vi "CoreVideo.vi"(11 "Cluster":T1) -> ()   [LabVIEW 2024]
uses:
  dacAquisition/#AquisitionLoopEnum.ctl
  <vilib>/vision/driver/IMAQdx.llb/IMAQdx Camera Control Mode.ctl
  <vilib>/vision/driver/NI_Vision_Acquisition_Software.lvlib
  <vilib>/vision/Image Controls.llb/IMAQ Image.ctl
  #VideoQueueElement.ctl
  #VisionProcessingEnum.ctl
  GUI/#GuiEnum.ctl
  GUI/#GuiQueueElement.ctl
  #QueueEnum.ctl
  Correlation/#CorrelationQueueElement.ctl
  <vilib>/userDefined/High Color/IMAQdx.ctl
  Core/#CoreQueues.ctl
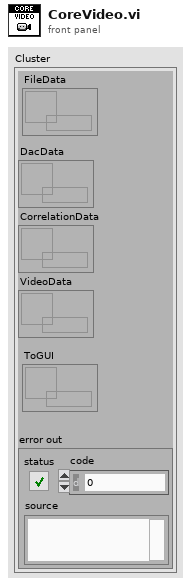
[diagram p1: front panel]
types:
  T1 = typedef "#CoreQueues.ctl" = cluster{"DacData":refnum<queue>, "CorrelationData":refnum<queue>, "VideoData":refnum<queue>, "error out":errorcluster, "ToGUI":refnum<queue>, "FileData":refnum<queue>}
  T2 = typedef "IMAQ Image.ctl" = refnum<image>
  T3 = typedef "IMAQdx.ctl" = refnum<k21>
  T4 = typedef "Image Type" = u32
  T5 = typedef "#VisionProcessingEnum.ctl" = enum16{"Init", "Processing", "ProcessingVision", "Close"}
  T6 = typedef "#AquisitionLoopEnum.ctl" = enum16{"Idle", "Init", "Aquisition", "End"}
  T7 = typedef "NI_Vision_Acquisition_Software.lvlib/IMAQdx Camera Control Mode.ctl" = enum32{"Controller", "Listener"}
  T8 = typedef "#VideoQueueElement.ctl" = cluster{"Image Out":T2, "current time":timestamp}
  T9 = typedef "#AntennaControlNumber.ctl" = enum16{"Ant1", "Ant2", "Ant3", "Ant4"}
  T10 = cluster{"Reverse fingers":bool, "SelectingButton":bool, "Antenna":T9, "TestVsion":bool, "Camera source":T3, "AntDistance [mm]":dbl}
  T11 = typedef "#GuiEnum.ctl" = enum16{"AudioData", "VisionDistances", "DacDistances", "CorrelationDistances", "Video", "FPS"}
  T12 = typedef "#GuiQueueElement.ctl" = cluster{"Enum":T11, "Variant":variant}
  T13 = typedef "#QueueEnum.ctl" = enum16{"Ant", "Video"}
  T14 = typedef "#CorrelationQueueElement.ctl" = cluster{"Enum":T13, "t0":timestamp, dbl[]}
  T15 = cluster{"Image Out":T2, "current time":timestamp}
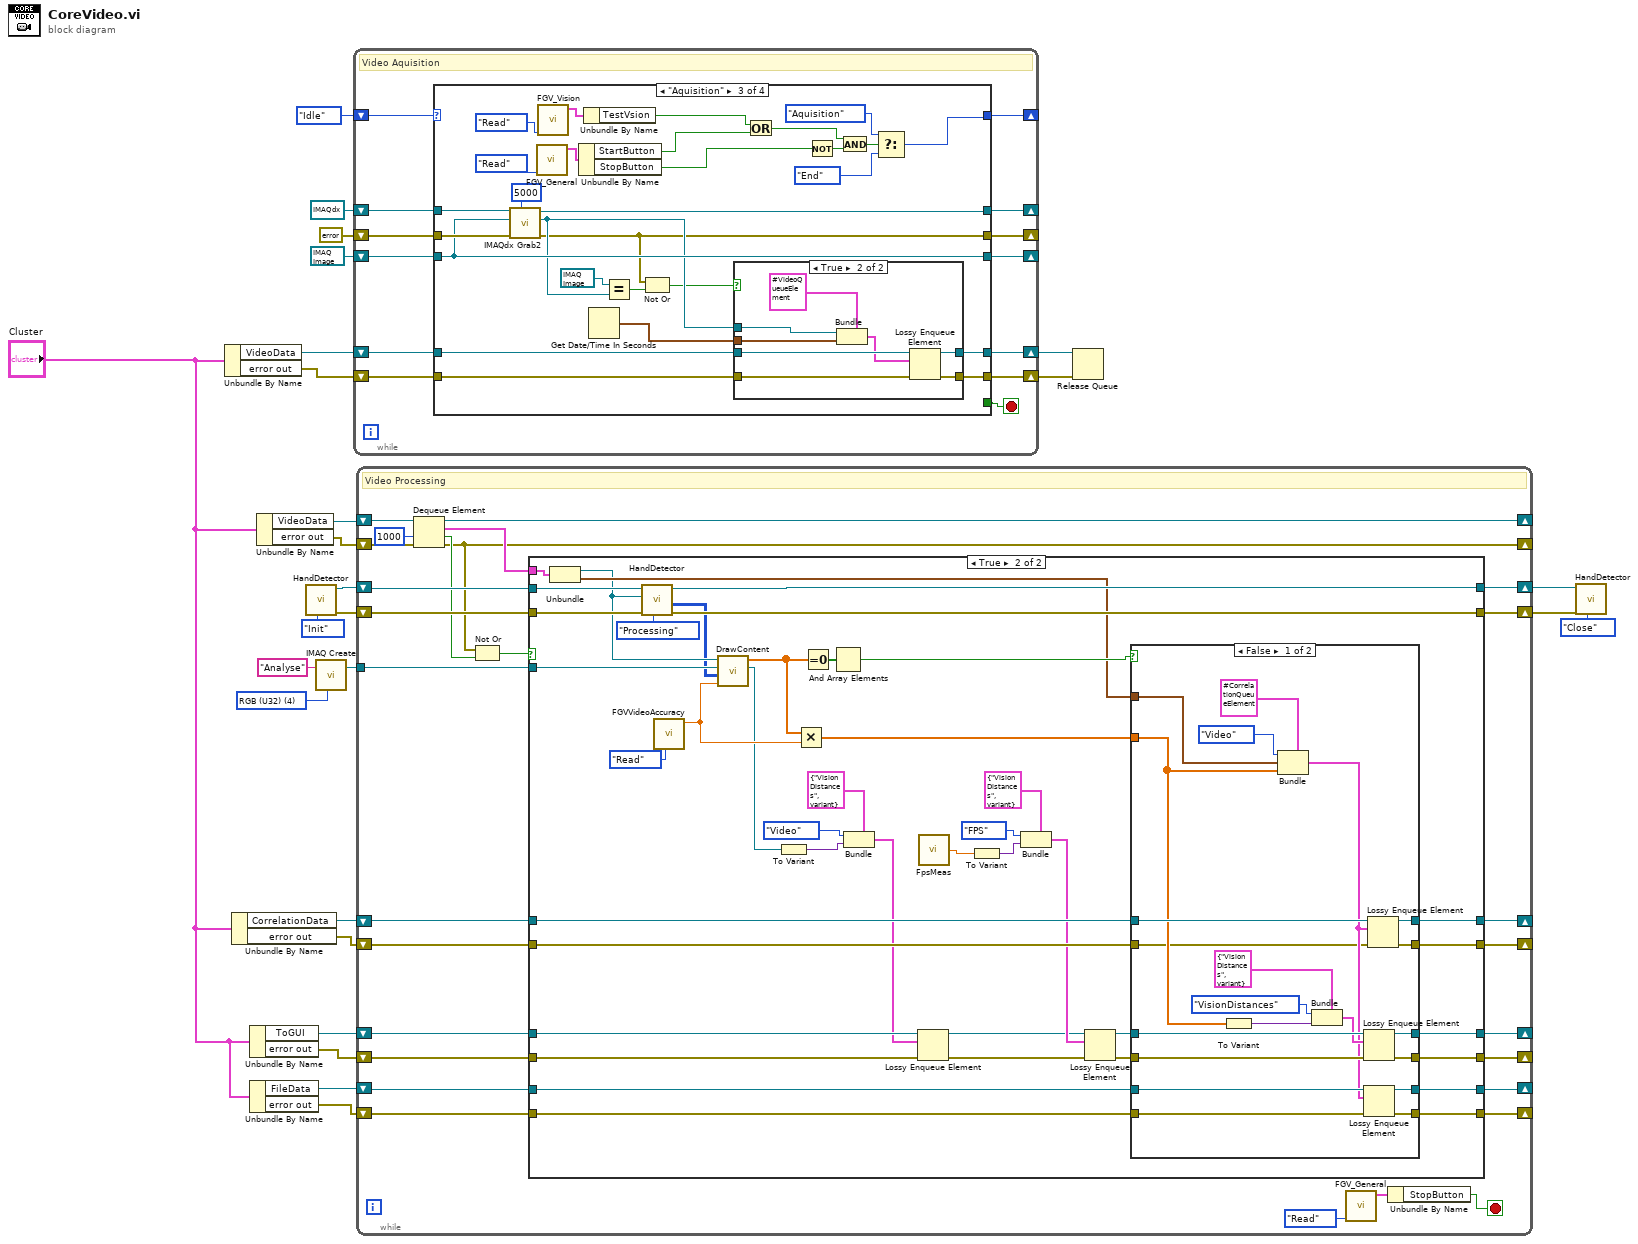
[diagram p0: block diagram]
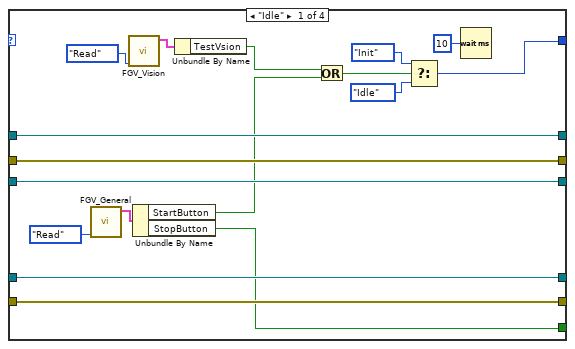
[diagram p4: hidden frame]
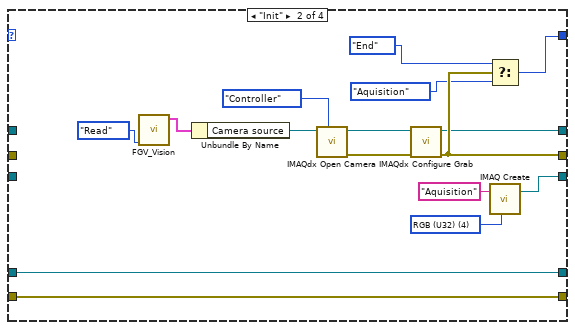
[diagram p5: hidden frame]
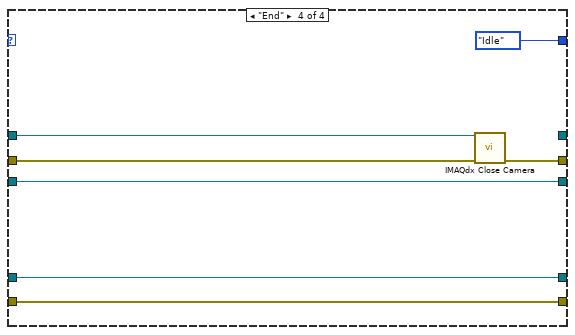
[diagram p7: hidden frame]
diagram:
  w12 = T4 4 items=["Grayscale (U8)", "Grayscale (I16)", "Grayscale (SGL)", "Complex (CSG)", "RGB (U32)", "HSL (U32)", "RGB (U64)", "Grayscale (U16)"] ("Image Type")
  n1 = Unbundle By Name("Cluster") -> ("VideoData"=w16:refnum<queue>, "error out"=w17:errorcluster)
  n2 = Unbundle By Name("Cluster") -> ("CorrelationData"=w23:refnum<queue>, "error out"=w24:errorcluster)
  n3 = Unbundle By Name("Cluster") -> ("ToGUI"=w25:refnum<queue>, "error out"=w26:errorcluster)
  n4 = Unbundle By Name("Cluster") -> ("FileData"=w3:refnum<queue>, "error out"=w2:errorcluster)
  n5 = Unbundle By Name("Cluster") -> ("VideoData"=w21:refnum<queue>, "error out"=w22:errorcluster)
  n6 = call "HandDetector.vi"("Enum"=#VisionProcessingEnum."Init") -> ("error out"=w10:errorcluster, "session out"=w9:refnum<k35>)  [unwired: 6 in, 3 out]
  n7 = call "IMAQ Create"("Image Name"="Analyse", "Image Type"=w12) -> ("New Image"=w13:T2)  [unwired: 3 in, 1 out]
  n8 = while {
    shift-right: [w39] -> _
    shift-left: T3 refnum ("Session Out") -> [w36]
    shift-right: [w38] -> _
    shift-left: errorcluster {"status"=FALSE, "code"=0, "source"=""} ("error out") -> [w37]
    shift-right: [w34] -> _
    shift-left: #AquisitionLoopEnum."Idle" -> [w35]
    shift-right: [w33] -> w14
    shift-left: w16 -> [w30]
    shift-right: [w32] -> w15
    shift-left: w17 -> [w31]
    shift-right: [w29] -> _
    shift-left: T2 refnum ("New Image") -> [w28]
    stop <- w27 stop-if-true
    # "Video Aquisition"
    n9 = case shown="\"Aquisition\"" w35 {
      tunnel: [w56 w57 w73 _] -> w39
      tunnel: [w55 w64 w83 w116] -> w38
      tunnel: w37 -> [w55 _ w100 w117]
      tunnel: w36 -> [w56 _ w74 w111]
      tunnel: [w51 w61 w94 #AquisitionLoopEnum."Idle"] -> w34
      tunnel: [w48 w69 w92 w114] -> w33
      tunnel: [w49 w68 w91 w113] -> w32
      tunnel: w31 -> [w49 w68 w90 w113]
      tunnel: w30 -> [w48 w69 w89 w114]
      tunnel: [w47 w67 w88 w112] -> w29
      tunnel: w28 -> [w47 _ w88 w112]
      tunnel: [w44 _ _ _] -> w27
      frame "Idle" {
        n10 = call "FGV_General.vi"("Type"=enum16{"Read", "Write"}."Read") -> ("GeneralIndicator"=w45:cluster{"StartButton":bool, "StopButton":bool})  [unwired: 10 in]
        n11 = call "FGV_Vision.vi"("Operation"=enum16{"Read", "Write"}."Read") -> ("OutVision"=w41:T10)  [unwired: 8 in]
        n12 = Unbundle By Name(w45) -> ("StartButton"=w43:bool, "StopButton"=w44:bool)
        n13 = Unbundle By Name(w41) -> ("TestVsion"=w40:bool)
        n14 = Or(x=w40, y=w43) -> (x .or. y?=w54:bool)
        n15 = Select(t=#AquisitionLoopEnum."Init", s=w54, f=#AquisitionLoopEnum."Idle") -> (s? t:f=w51:T6)
        n16 = Wait (ms)(milliseconds to wait=u32 10) -> ()  [unwired: 1 out]
      }
      frame "Init" {
        w65 = T4 4 items=["Grayscale (U8)", "Grayscale (I16)", "Grayscale (SGL)", "Complex (CSG)", "RGB (U32)", "HSL (U32)", "RGB (U64)", "Grayscale (U16)"] ("Image Type")
        n17 = call "FGV_Vision.vi"("Operation"=enum16{"Read", "Write"}."Read") -> ("OutVision"=w59:T10)  [unwired: 8 in]
        n18 = Unbundle By Name(w59) -> ("Camera source"=w58:T3)
        n19 = call <vilib>:"IMAQdx Open Camera.vi"("Camera Control Mode"=IMAQdx_Camera_Control_Mode."Controller", "Session In"=w58) -> ("error out"=w70:errorcluster, "Session Out"=w72:T3)  [unwired: 8 in]
        n20 = call <vilib>:"IMAQdx Configure Grab.vi"("error in"=w70, "Session In"=w72) -> ("error out"=w64:errorcluster, "Session Out"=w57:T3)  [unwired: 8 in]
        n21 = Select(t=#AquisitionLoopEnum."End", s=w64, f=#AquisitionLoopEnum."Aquisition") -> (s? t:f=w61:T6)
        n22 = call "IMAQ Create"("Image Name"="Aquisition", "Image Type"=w65) -> ("New Image"=w67:T2)  [unwired: 3 in, 1 out]
      }
      frame "Aquisition" {
        n23 = call <vilib>:"IMAQdx Grab2.vi"("Timeout (ms)"=5000, "error in"=w100, "Image In"=w88, "Session In"=w74) -> ("error out"=w83:errorcluster, "Image Out"=w86:T2, "Session Out"=w73:T3)  [unwired: 4 in, 1 out]
        n24 = call "FGV_General.vi"("Type"=enum16{"Read", "Write"}."Read") -> ("GeneralIndicator"=w80:cluster{"StartButton":bool, "StopButton":bool})  [unwired: 10 in]
        n25 = call "FGV_Vision.vi"("Operation"=enum16{"Read", "Write"}."Read") -> ("OutVision"=w76:T10)  [unwired: 8 in]
        n26 = Unbundle By Name(w80) -> ("StartButton"=w78:bool, "StopButton"=w79:bool)
        n27 = Unbundle By Name(w76) -> ("TestVsion"=w75:bool)
        n28 = Get Date/Time In Seconds() -> (seconds since 1Jan1904=w82:timestamp)
        n29 = Equal?(x=T2 refnum ("Image Out"), y=w86) -> (x = y?=w84:bool)
        n30 = Not Or(1:w84, 2:w83) -> (0:w85:bool)
        n31 = case shown="True" w85 {
          tunnel: [w102 w110] -> w92
          tunnel: [w101 w109] -> w91
          tunnel: w90 -> [w101 w103]
          tunnel: w89 -> [w102 w108]
          tunnel: w86 -> [_ w107]
          tunnel: w82 -> [_ w106]
          frame False {
          }
          frame True {
            n32 = Bundle(cluster=T8 {"Image Out"=refnum, "current time"=timestamp(0 s since 1904-01-01)}, "Image Out"=w107, "current time"=w106) -> (w104:T8)
            n33 = Lossy Enqueue Element(queue=w108, element=w104, error in (no error)=w103) -> (queue out=w110:refnum<queue>, error out=w109:errorcluster)  [unwired: 2 out]
          }
        }
        n34 = Or(x=w75, y=w78) -> (x .or. y?=w97:bool)
        n35 = Not(x=w79) -> (.not. x?=w99:bool)
        n36 = And(x=w97, y=w99) -> (x .and. y?=w98:bool)
        n37 = Select(t=#AquisitionLoopEnum."Aquisition", s=w98, f=#AquisitionLoopEnum."End") -> (s? t:f=w94:T6)
      }
      frame "End" {
        n38 = call <vilib>:"IMAQdx Close Camera.vi"("error in"=w117, "Session In"=w111) -> ("error out"=w116:errorcluster)  [unwired: 9 in]
      }
    }
  }
  n39 = while {
    shift-right: [w143] -> _
    shift-left: w21 -> [w145]
    shift-right: [w133] -> _
    shift-left: w22 -> [w144]
    shift-right: [w142] -> w7
    shift-left: w9 -> [w140]
    shift-right: [w134] -> w8
    shift-left: w10 -> [w141]
    tunnel: w13 -> [w137]
    shift-right: [w130] -> _
    shift-left: w24 -> [w131]
    shift-right: [w129] -> _
    shift-left: w23 -> [w132]
    shift-right: [w125] -> _
    shift-left: w25 -> [w124]
    shift-right: [w122] -> _
    shift-left: w26 -> [w123]
    shift-right: [w121] -> _
    shift-left: w3 -> [w120]
    shift-right: [w118] -> _
    shift-left: w2 -> [w119]
    stop <- w126 stop-if-true
    # "Video Processing"
    n40 = Dequeue Element(queue=w145, timeout in ms (-1)=1000, error in (no error)=w144) -> (queue out=w143:refnum<queue>, element=w139:T15, timed out?=w136:bool, error out=w133:errorcluster)
    n41 = Not Or(1:w136, 2:w133) -> (0:w135:bool)
    n42 = case shown="True" w135 {
      tunnel: [w152 w192] -> w142
      tunnel: [w153 w193] -> w134
      tunnel: w141 -> [w153 w194]
      tunnel: w140 -> [w152 w195]
      tunnel: w139 -> [_ w189]
      tunnel: w137 -> [_ w181]
      tunnel: w132 -> [w151 w187]
      tunnel: w131 -> [w150 w186]
      tunnel: [w150 w184] -> w130
      tunnel: [w151 w185] -> w129
      tunnel: [w149 w170] -> w125
      tunnel: w124 -> [w149 w165]
      tunnel: w123 -> [w148 w164]
      tunnel: [w148 w167] -> w122
      tunnel: [w147 w157] -> w121
      tunnel: w120 -> [w147 w156]
      tunnel: w119 -> [w146 w155]
      tunnel: [w146 w154] -> w118
      frame False {
      }
      frame True {
        n43 = Unbundle(w189) -> ("Image Out"=w182:T2, "current time"=w188:timestamp)
        n44 = call "HandDetector.vi"("Enum"=#VisionProcessingEnum."Processing", "error in (no error)"=w194, "Image"=w182, "session in"=w195) -> ("error out"=w193:errorcluster, "Landmarkers coords"=w180:u32[][], "session out"=w192:refnum<k35>)  [unwired: 3 in, 2 out]
        n45 = call "FGVVideoAccuracy.vi"("Operation"=enum16{"Read", "Write"}."Read") -> ("VideoAccuracy"=w171:dbl)  [unwired: 10 in]
        n46 = call "DrawContent.vi"("In Image"=w182, "New Image"=w181, "Normalized Landmakers"=w180, "VideoAccuracy [mm/px]"=w171) -> ("Distances"=w179:dbl[], "Out Image"=w158:T2)  [unwired: 5 in]
        n47 = To Variant(anything=w158) -> (Variant=w159:variant)
        n48 = Multiply(x=w179, y=w171) -> (x*y=w183:dbl[])
        n49 = Equal To 0?(x=w179) -> (x = 0?=w178:bool[])
        n50 = And Array Elements(Boolean array=w178) -> (logical AND=w190:bool)
        n51 = Bundle(cluster=T12 {"Enum"=enum."VisionDistances", "Variant"=variant} ("element"), "Enum"=#GuiEnum."Video", "Variant"=w159) -> (w160:T12)
        n52 = Lossy Enqueue Element(queue=w165, element=w160, error in (no error)=w164) -> (queue out=w166:refnum<queue>, error out=w163:errorcluster)  [unwired: 2 out]
        n53 = call "FpsMeas.vi"() -> ("FPS"=w173:dbl)  [unwired: 2 in]
        n54 = To Variant(anything=w173) -> (Variant=w174:variant)
        n55 = Bundle(cluster=T12 {"Enum"=enum."VisionDistances", "Variant"=variant} ("element"), "Enum"=#GuiEnum."FPS", "Variant"=w174) -> (w175:T12)
        n56 = Lossy Enqueue Element(queue=w166, element=w175, error in (no error)=w163) -> (queue out=w169:refnum<queue>, error out=w168:errorcluster)  [unwired: 2 out]
        n57 = case shown="False" w190 {
          tunnel: w183 -> [w202 _]
          tunnel: w188 -> [w216 _]
          tunnel: w187 -> [w215 w222]
          tunnel: w186 -> [w196 w221]
          tunnel: [w214 w222] -> w185
          tunnel: [w213 w221] -> w184
          tunnel: [w207 w220] -> w170
          tunnel: w169 -> [w210 w220]
          tunnel: w168 -> [w209 w219]
          tunnel: [w208 w219] -> w167
          tunnel: [w201 w218] -> w157
          tunnel: w156 -> [w200 w218]
          tunnel: w155 -> [w199 w217]
          tunnel: [w198 w217] -> w154
          frame False {
            n58 = To Variant(anything=w202) -> (Variant=w203:variant)
            n59 = Bundle(cluster=T14 {"Enum"=enum."Video", "t0"=timestamp(0 s since 1904-01-01), []}, "Enum"=#QueueEnum."Video", "t0"=w216, w202) -> (w197:T14)
            n60 = Bundle(cluster=T12 {"Enum"=enum."VisionDistances", "Variant"=variant} ("element"), "Enum"=#GuiEnum."VisionDistances", "Variant"=w203) -> (w204:T12)
            n61 = Lossy Enqueue Element(queue=w210, element=w204, error in (no error)=w209) -> (queue out=w207:refnum<queue>, error out=w208:errorcluster)  [unwired: 2 out]
            n62 = Lossy Enqueue Element(queue=w200, element=w197, error in (no error)=w199) -> (queue out=w201:refnum<queue>, error out=w198:errorcluster)  [unwired: 2 out]
            n63 = Lossy Enqueue Element(queue=w215, element=w197, error in (no error)=w196) -> (queue out=w214:refnum<queue>, error out=w213:errorcluster)  [unwired: 2 out]
          }
          frame True {
          }
        }
      }
    }
    n64 = call "FGV_General.vi"("Type"=enum16{"Read", "Write"}."Read") -> ("GeneralIndicator"=w127:cluster{"StartButton":bool, "StopButton":bool})  [unwired: 10 in]
    n65 = Unbundle By Name(w127) -> ("StopButton"=w126:bool)
  }
  n66 = Release Queue(queue=w14, error in (no error)=w15) -> ()  [unwired: 1 in, 3 out]
  n67 = call "HandDetector.vi"("Enum"=#VisionProcessingEnum."Close", "error in (no error)"=w8, "session in"=w7) -> ()  [unwired: 4 in, 5 out]
